vi "DLPVA-100-B_&_F.vi"(0 "Index":i32, 5 "Gain_1 i":bool, 7 "Gain_2 i":bool, 9 "AC/DC":bool=TRUE, 11 "Filter":bool=TRUE) -> (4 "Gain (dB)":dbl, 6 "Gain_1o":bool, 8 "Gain_2 o":bool, 10 "AC/DC o":bool=TRUE, 15 "Filter o":bool=TRUE)   [LabVIEW 2010]
uses:
  <userlib>/FEMTO/Control/Set_Bandwidth_DLPVA-Series.vi
  <userlib>/FEMTO/Control/Set_Gain_DLPVA-100-B&F_Series.vi
  <userlib>/FEMTO/FEMTO_LUCI-10.lvlib
panel:
  in  "Info":bool
  out "Gain_Stages 2":bool[](array[boolean])=[FALSE, FALSE, FALSE, TRUE, FALSE, FALSE, FALSE, FALSE, FALSE, FALSE, FALSE, FALSE, FALSE, FALSE, FALSE, FALSE, FALSE, FALSE, FALSE, FALSE, FALSE, FALSE, FALSE, FALSE, FALSE, FALSE, FALSE, FALSE, FALSE, FALSE, FALSE, FALSE]
  out "Overload":bool
  in  "stop":bool
  out "LED":bool
  in  "Check LUCI":bool
  out "String_Product":string
  in  "Product_String":bool
  # "Remote Control LUCI-10 DLPVA-100"
  # "DLPVA-100-B & F"
  # "Configuration"
  # "Gain Setting"
  # "Overal Gain"
  # "80 dB"
  # "60 dB"
  # "Device Information"
  # "40 dB"
  # "20 dB"
  # "40 dB"
  # "20 dB"
  # "0 dB"
  # "0 dB"
  # "Filter"
  # "Coupling"
  # "1 kHz"
  # "AC"
  # "100 kHz"
  # "DC"
  # "Sophisticated Tools for Signal Recovery"
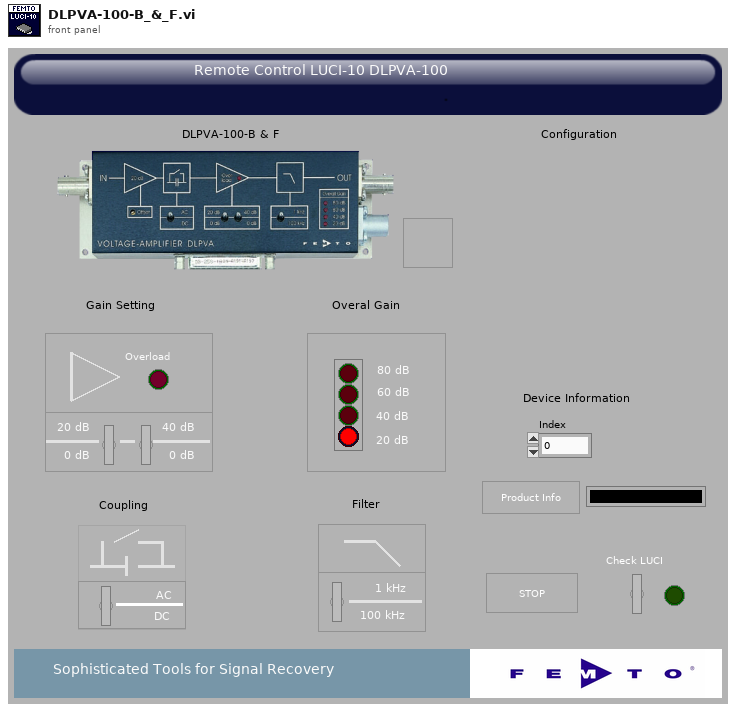
[diagram p1: front panel]
types:
  T1 = enum16{"DDPCA-300", "DLPCA-200", "DHPCA-100", "OE-200", "LIA-MV-150-S", "LIA-MV-150-D", "LIA-MV-200-L", "LIA-MV-200-H", "LIA-MVD-200-L", "LIA-MVD-200-H", "DLPVA-100-BUN-S", "DLPVA-100-BLN-S", "DLPVA-100-B-S", "DLPVA-100-B-D", "DLPVA-100-F-S", "DLPVA-100-F-D", "DHPVA-100", "DHPVA-200", "DUPVA-1-60", "DUPVA-1-70"}
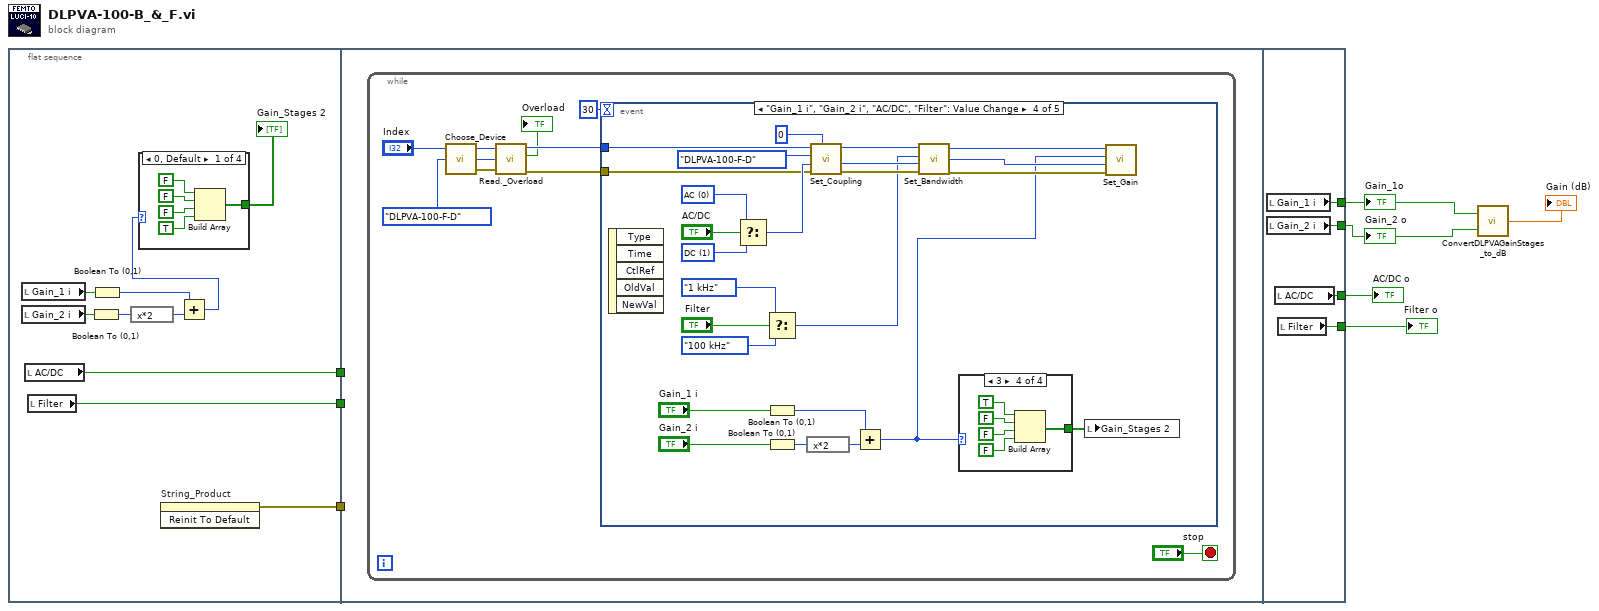
[diagram p0: block diagram]
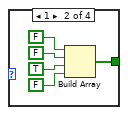
[diagram p2: hidden frame]
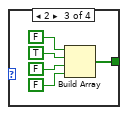
[diagram p3: hidden frame]
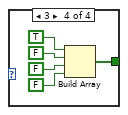
[diagram p4: hidden frame]
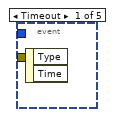
[diagram p5: hidden frame]
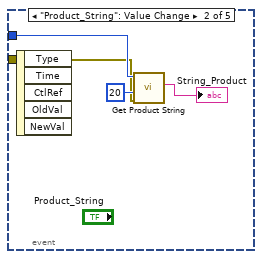
[diagram p6: hidden frame]
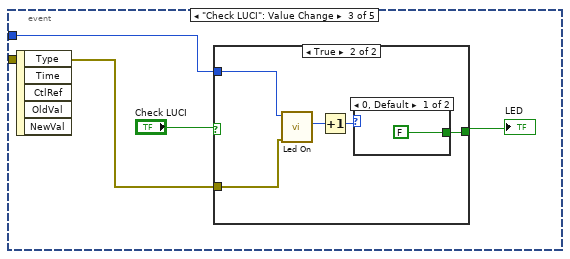
[diagram p7: hidden frame]
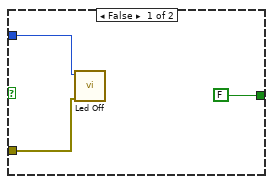
[diagram p8: hidden frame]
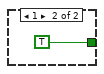
[diagram p9: hidden frame]
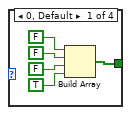
[diagram p10: hidden frame]
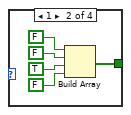
[diagram p11: hidden frame]
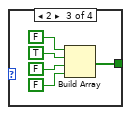
[diagram p12: hidden frame]
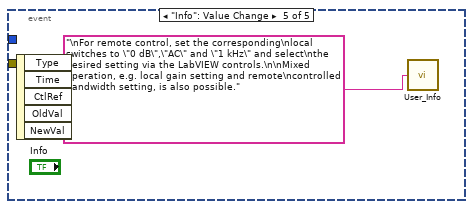
[diagram p13: hidden frame]
diagram:
  n1 = flat-sequence {
    tunnel: [w12] -> w8
    tunnel: [w11] -> w5
    tunnel: [w10] -> w4
    tunnel: w8 -> [_]
    tunnel: w5 -> [_]
    tunnel: w4 -> [_]
    tunnel: [w116] -> w3
    tunnel: [w115] -> w2
    tunnel: [w114] -> w6
    tunnel: [w113] -> w7
    frame #0 {
      n2 = local read "Gain_1 i"() -> (w18:bool)
      n3 = local read "Gain_2 i"() -> (w17:bool)
      n4 = local read "AC/DC"() -> (w11:bool)
      n5 = local read "Filter"() -> (w10:bool)
      n6 = Boolean To (0,1)(Boolean=w17) -> (0, 1=w16:i16)
      n7 = Boolean To (0,1)(Boolean=w18) -> (0, 1=w14:i16)
      n8 = expression code="x*2"(w16) -> (w15:i16)
      n9 = invoke on="String_Product" class="Str" method="Reinit To Default"() -> (error out=w12:errorcluster)  [unwired: 3 in, 2 out]
      n10 = Add(x=w14, y=w15) -> (x+y=w9:i16)
      n11 = case shown="0, Default" w9 {
        tunnel: [w19 w24 w29 w34] -> w13
        frame 0, Default {
          n12 = Build Array(FALSE ("new element/subarray"), FALSE ("new element/subarray"), FALSE ("new element/subarray"), TRUE ("new element/subarray")) -> (w19:bool[])
        }
        frame 1 {
          n13 = Build Array(FALSE ("new element/subarray"), FALSE ("new element/subarray"), TRUE ("new element/subarray"), FALSE ("new element/subarray")) -> (w24:bool[])
        }
        frame 2 {
          n14 = Build Array(FALSE ("new element/subarray"), TRUE ("new element/subarray"), FALSE ("new element/subarray"), FALSE ("new element/subarray")) -> (w29:bool[])
        }
        frame 3 {
          n15 = Build Array(TRUE ("new element/subarray"), FALSE ("new element/subarray"), FALSE ("new element/subarray"), FALSE ("new element/subarray")) -> (w34:bool[])
        }
      }
      "Gain_Stages 2" <- w13
    }
    frame #1 {
      n16 = while {
        stop <- "stop" stop-if-true
        n17 = call <userlib>:"Choose_Device.vi"("Choose_Device"=T1."DLPVA-100-F-D", "Index"="Index") -> ("error out"=w43:errorcluster, "Device_type"=w40:T1, "Index_Out"=w45:i32)  [unwired: 1 in]
        n18 = call <userlib>:"Read._Overload.vi"("Index"=w45, "Choose_Device"=w40, "error in (no error)"=w43) -> ("Index_Out"=w44:i32, "Overload"=→"Overload":bool, "error out"=w42:errorcluster)  [unwired: 1 out]
        n19 = event shown="[3] \"Gain_1 i\", \"Gain_2 i\", \"AC/DC\", \"Filter\": Value Change" {
          selector: _ -> [_ _ _ _ _]
          dyn-events: _ -> [_ _ _ _ _]
          timeout: 30 -> [_ _ _ _ _]
          tunnel: w42 -> [_ w50 w55 w72 _]
          tunnel: w44 -> [_ w52 w56 w90 _]
          event Timeout {
            n20 = event-data() -> ()  [unwired: 3 out]
          }
          event "Product_String": Value Change {
            n21 = event-data() -> ()  [unwired: 6 out]
            n22 = call <userlib>:"Get Product String.vi"("error in (no error)"=w50, "size"=20, "index"=w52) -> ("string out"=→"String_Product":string)  [unwired: 8 out]
          }
          event "Check LUCI": Value Change {
            n23 = event-data() -> ()  [unwired: 6 out]
            n24 = case shown="True" "Check LUCI" {
              tunnel: w56 -> [w59 w64]
              tunnel: w55 -> [w58 w63]
              tunnel: [FALSE w60] -> w53
              frame False {
                n25 = call <userlib>:"Led Off.vi"("error in (no error)"=w58, "index"=w59) -> ()  [unwired: 10 out]
              }
              frame True {
                n26 = call <userlib>:"Led On.vi"("error in (no error)"=w63, "index"=w64) -> ("function_return"=w62:i32)  [unwired: 9 out]
                n27 = Increment(x=w62) -> (x+1=w61:i32)
                n28 = case shown="0, Default" w61 {
                  tunnel: [FALSE TRUE] -> w60
                  frame 0, Default {
                  }
                  frame 1 {
                  }
                }
              }
            }
            "LED" <- w53
          }
          event "Gain_1 i", "Gain_2 i", "AC/DC", "Filter": Value Change {
            w76 = u16 1 items=["AC", "DC"] ("Set Coupling")
            w77 = u16 0 items=["AC", "DC"] ("Set Coupling")
            n29 = event-data() -> ()  [unwired: 6 out]
            n30 = Select(t=w77, s="AC/DC", f=w76) -> (s? t:f=w73:u16)
            n31 = Select(t=enum16{"1 kHz", "100 kHz"}."1 kHz" ("Bandwidth"), s="Filter", f=enum16{"1 kHz", "100 kHz"}."100 kHz" ("Bandwidth")) -> (s? t:f=w83:enum16{"1 kHz", "100 kHz"})
            n32 = Boolean To (0,1)(Boolean="Gain_1 i") -> (0, 1=w70:i16)
            n33 = Boolean To (0,1)(Boolean="Gain_2 i") -> (0, 1=w82:i16)
            n34 = expression code="x*2"(w82) -> (w81:i16)
            n35 = call <userlib>:"Set_Coupling.vi"("Status"=0, "error in (no error)"=w72, "Set Coupling"=w73, "Choose_Device"=T1."DLPVA-100-F-D", "Index"=w90) -> ("error out"=w85:errorcluster, "Status_out"=w86:i32, "Index_Out"=w87:i32)  [unwired: 1 out]
            n36 = Add(x=w70, y=w81) -> (x+y=w71:i16)
            n37 = call-poly <userlib>:"Set_Bandwidth.vi"("error in"=w85, "Status"=w86, "Bandwidth"=w83, "index"=w87) -> ("error out"=w78:errorcluster, "Status_out"=w79:i32, "index_out"=w80:i32)
            n38 = case shown="3" w71 {
              tunnel: [w92 w97 w102 w107] -> w67
              frame 0, Default {
                n39 = Build Array(FALSE ("new element/subarray"), FALSE ("new element/subarray"), FALSE ("new element/subarray"), TRUE ("new element/subarray")) -> (w92:bool[])
              }
              frame 1 {
                n40 = Build Array(FALSE ("new element/subarray"), FALSE ("new element/subarray"), TRUE ("new element/subarray"), FALSE ("new element/subarray")) -> (w97:bool[])
              }
              frame 2 {
                n41 = Build Array(FALSE ("new element/subarray"), TRUE ("new element/subarray"), FALSE ("new element/subarray"), FALSE ("new element/subarray")) -> (w102:bool[])
              }
              frame 3 {
                n42 = Build Array(TRUE ("new element/subarray"), FALSE ("new element/subarray"), FALSE ("new element/subarray"), FALSE ("new element/subarray")) -> (w107:bool[])
              }
            }
            n43 = local write "Gain_Stages 2"(w67) -> ()
            n44 = call-poly <userlib>:"Set_Gain.vi"("error in"=w78, "Status"=w79, "Gain [dB]"=w71, "index"=w80) -> ()  [unwired: 3 out]
          }
          event "Info": Value Change {
            n45 = event-data() -> ()  [unwired: 6 out]
            n46 = call <userlib>:"User_Info.vi"("String"="\nFor remote control, set the corresponding\nlocal switches to \"0 dB\",\"AC\" and \"1 kHz\" and select\nthe desired setting via the LabVIEW controls.\n\nMixed operation, e.g. local gain setting and remote\ncontrolled bandwidth setting, is also possible.") -> ()  [unwired: 1 out]
          }
        }
      }
    }
    frame #2 {
      n47 = local read "Gain_1 i"() -> (w116:bool)
      n48 = local read "Gain_2 i"() -> (w115:bool)
      n49 = local read "AC/DC"() -> (w114:bool)
      n50 = local read "Filter"() -> (w113:bool)
    }
  }
  n51 = call "ConvertDLPVAGainStages_to_dB.vi"("Gain_2 i"=w2, "Gain_1 i"=w3) -> ("Gain (dB)"=→"Gain (dB)":dbl)
  "Gain_1o" <- w3
  "Gain_2 o" <- w2
  "AC/DC o" <- w6
  "Filter o" <- w7
